vi "ComPort_Replace.vi"(11 "Path":path) -> ()   [LabVIEW 2024]
panel:
  out "text":string
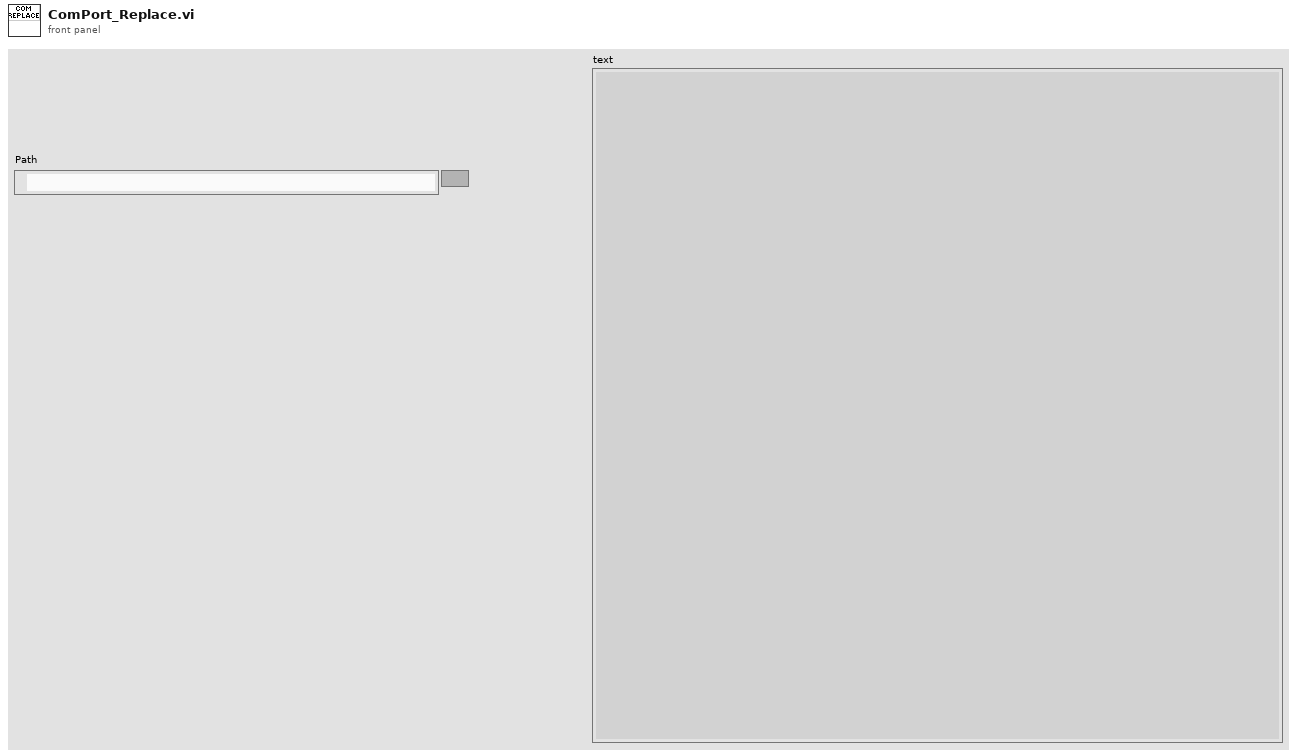
[diagram p1: front panel]
types:
  T1 = enum16{"open", "replace", "create", "open or create", "replace or create", "replace or create with confirmation"}
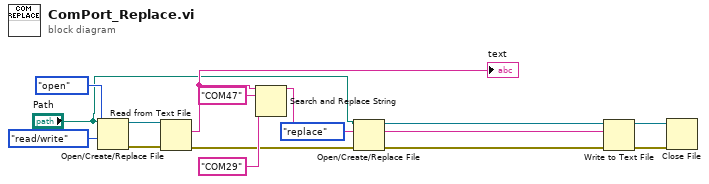
[diagram p0: block diagram]
diagram:
  n1 = Open/Create/Replace File(file path (use dialog)="Path", operation (0:open)=T1."open", access (0:read/write)=enum16{"read/write", "read-only", "write-only"}."read/write") -> (refnum out=w13:refnum<file>, error out=w14:errorcluster)  [unwired: 3 in, 1 out]
  n2 = Read from Text File(file (use dialog)=w13, error in=w14) -> (text=w7:string, error out=w4:errorcluster)  [unwired: 2 in, 2 out]
  "text" <- w7
  n3 = Search and Replace String(input string=w7, search string="COM47", replace string="COM29" ("replace string (\"\")")) -> (result string=w10:string)  [unwired: 5 in, 3 out]
  n4 = Open/Create/Replace File(file path (use dialog)="Path", error in=w4, operation (0:open)=T1."replace") -> (refnum out=w1:refnum<file>)  [unwired: 3 in, 2 out]
  n5 = Write to Text File(file (use dialog)=w1, text=w10, error in=w4) -> (refnum out=w9:refnum<file>, error out=w8:errorcluster)  [unwired: 1 in, 1 out]
  n6 = Close File(refnum=w9, error in=w8) -> ()  [unwired: 2 out]
